vi "Get Max 1D 3p.vi"(2 "CrossCorrelation":dbl[](array[numeric]) format="%.2f") -> (0 "Position":dbl format="%.4f")   [LabVIEW 2011, in "OfflineTracker.lvlib"]
uses:
  OfflineTracker.lvlib
panel:
  in  "Case Constant\n(See Context Help)":enum16{"3points", "5points"}(ring)=enum."5points"
  out "Waveform Graph":dbl[][](graph)
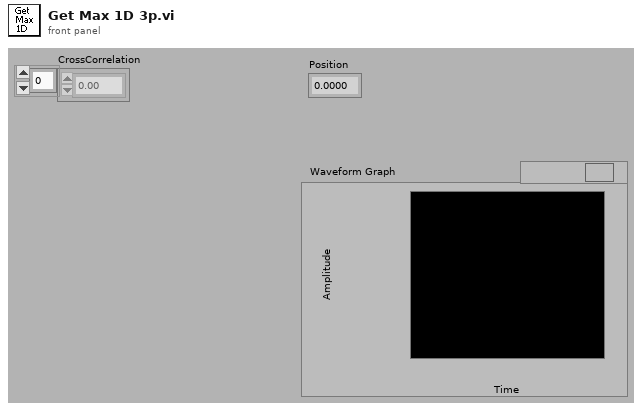
[diagram p1: front panel]
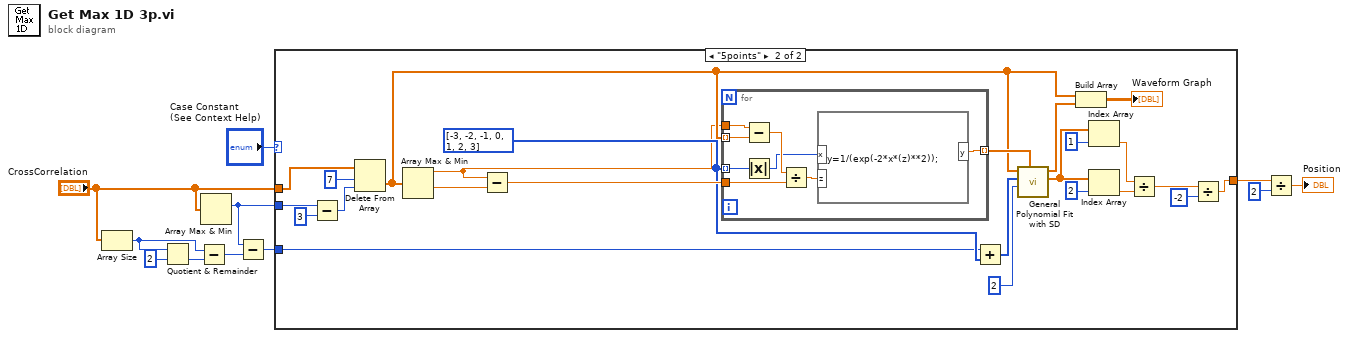
[diagram p0: block diagram]
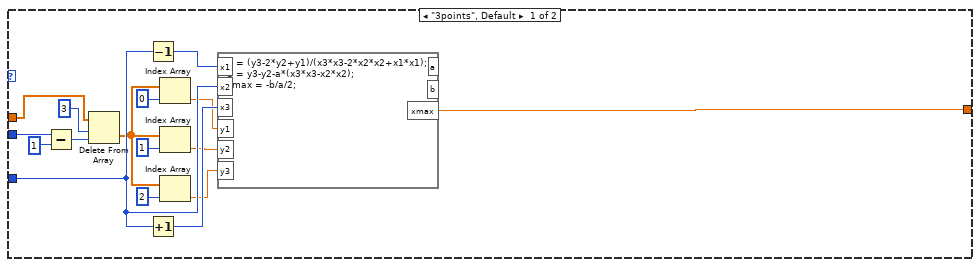
[diagram p2: hidden frame]
diagram:
  n1 = Array Size(array="CrossCorrelation") -> (size(s)=w6:i32)
  n2 = Quotient & Remainder(x=w6, y=2) -> (floor(x/y)=w9:i32)  [unwired: 1 out]
  n3 = Subtract(x=w6, y=w9) -> (x-y=w1:i32)
  n4 = Array Max & Min(array="CrossCorrelation") -> (max index (indices)=w4:i32)  [unwired: 3 out]
  n5 = Subtract(x=w4, y=w1) -> (x-y=w8:i32)
  n6 = case shown="\"5points\"" "Case Constant\n(See Context Help)" {
    tunnel: w8 -> [w26 w31]
    tunnel: [w18 w30] -> w2
    tunnel: w4 -> [w14 w32]
    tunnel: "CrossCorrelation" -> [w13 w33]
    frame "3points", Default {
      n7 = Subtract(x=w14, y=1) -> (x-y=w17:i32)
      n8 = Delete From Array(array=w13, length=3, index=w17) -> (deleted portion=w12:dbl[])  [unwired: 1 out]
      n9 = Decrement(x=w26) -> (x-1=w27:i32)
      n10 = Increment(x=w26) -> (x+1=w25:i32)
      n11 = Index Array(array=w12, index=0) -> (element=w24:dbl)
      n12 = Index Array(array=w12, index=1) -> (element=w19:dbl)
      n13 = Index Array(array=w12, index=2) -> (element=w20:dbl)
      n14 = formula code="a = (y3-2*y2+y1)/(x3*x3-2*x2*x2+x1*x1);\nb = y3-y2-a*(x3*x3-x2*x2);\nxmax = -b/a/2;"("x1"=w27, "x2"=w26, "x3"=w25, "y1"=w24, "y2"=w19, "y3"=w20) -> ("xmax"=w18:dbl)  [unwired: 2 out]
    }
    frame "5points" {
      w34 = i8[] [-3, -2, -1, 0, 1, 2, 3]
      n15 = Subtract(x=w32, y=3) -> (x-y=w50:i32)
      n16 = Delete From Array(array=w33, length=7, index=w50) -> (deleted portion=w37:dbl[])  [unwired: 1 out]
      n17 = Array Max & Min(array=w37) -> (max value=w29:dbl, min value=w36:dbl)  [unwired: 2 out]
      n18 = Subtract(x=w29, y=w36) -> (x-y=w35:dbl)
      n19 = for {
        tunnel: [w59] -> w51 mode=indexing
        tunnel: w37 -> [w53] mode=indexing
        tunnel: w35 -> [w57]
        tunnel: w34 -> [w55] mode=indexing
        tunnel: w29 -> [w52]
        n20 = Subtract(x=w52, y=w53) -> (x-y=w58:dbl)
        n21 = Absolute Value(x=w55) -> (abs(x)=w54:i8)
        n22 = Divide(x=w58, y=w57) -> (x/y=w56:dbl)
        n23 = formula code="y=1/(exp(-2*x*(z)**2));"("z"=w56, "x"=w54) -> ("y"=w59:dbl)
      }
      n24 = Add(x=w31, y=w34) -> (x+y=w47:i32[])
      n25 = call "General Polynomial Fit with SD.vi"("Standard Deviation"=w51, "polynomial order"=2, "X Values"=w47, "Y Values"=w37) -> ("Polynomial Fit Coefficients"=w43:dbl[], "Best Polynomial Fit"=w38:dbl[])  [unwired: 1 in, 2 out]
      n26 = Build Array(w37, w38) -> (→"Waveform Graph":dbl[][])
      n27 = Index Array(array=w43, index=1) -> (element=w42:dbl)
      n28 = Index Array(array=w43, index=2) -> (element=w41:dbl)
      n29 = Divide(x=w42, y=w41) -> (x/y=w40:dbl)
      n30 = Divide(x=w40, y=i8 -2) -> (x/y=w30:dbl)
    }
  }
  n31 = Divide(x=w2, y=i8 2) -> (x/y=→"Position":dbl)
